vi "Target Vision Processing.vi"(4 "error in (no error)":errorcluster, 7 "Target Camera Image Size":T3=enum."160x120") -> ()   [LabVIEW 2015]
uses:
  Vision Support Code/Camera Types.ctl
  <vilib>/Rock Robotics/WPI/Camera/WPI_CameraImageSize.ctl
  <vilib>/Rock Robotics/WPI/Camera/WPI_CameraWhite Balance Values.ctl
  <vilib>/Rock Robotics/WPI/Camera/WPI_CameraExposure Values.ctl
  <vilib>/Rock Robotics/WPI/Camera/WPI_CameraFrameRate.ctl
  Robot Global Data.vi
  <vilib>/vision/NI_Vision_Development_Module.lvlib
panel:
  out "Highest Avg Score":dbl=93.76490466950331
  out "Detected Targets":T1(array[cluster])=[{"Distance (ft)"=10.934953821756244, "Center"={-0.006249999999999922, 0.175}, "Normalized Rect"={"Numeric"=-0.16249999999999998, "Numeric 2"=0.2833333333333333, "Numeric 3"=0.15000000000000013, "Numeric 5"=0.06666666666666665}}] {"Normalized Rect"."Numeric 5" format="%#_2g"; "Normalized Rect"."Numeric 3" format="%#_2g"; "Normalized Rect"."Numeric 2" format="%#_2g"; "Normalized Rect"."Numeric" format="%#_2g"}
  out "Sorted Particle Scores":T2(array[cluster])=[{"Rectangle px"={"Numeric"=67.0, "Numeric 2"=43.0, "Numeric 3"=92.0, "Numeric 5"=56.0}, "Aspect Ratio"=79.80769230769232, "Area to CH"=82.27848101265822, "X"=100.0, "Y"=100.0, "Moment Factor"=94.26815936617268}] {"Moment Factor" format="%#_3g"; "Aspect Ratio" format="%#_3g"; "Area to CH" format="%#_3g"; "X" format="%#_3g"; "Y" format="%#_3g"}
  in  "Display Original":bool=TRUE
  in  "Display Mask":bool=TRUE
  in  "Emphasize Limit Tests":bool=TRUE
  in  "Camera Type":T4=enum."MS HD3000 square"
  in  "Aspect Fudge Factor":dbl=1.0
  in  "Score Threshold":dbl=75.0
  out "Qualified Particles":i32=3
  in  "LED Color":T5={"Hue"={70.0, 10.0}, "Sat"={6.071428571428582, 255.0}, "Val"={127.5, 255.0}} {"Hue" scale=0.0..255.0 scale format="%#_3g"}
  out "Masked":T6(plugin-control)
  out "Original Image":T6(plugin-control)
  # "TARGET VISION PROCESSING.VI"
  # "This is only the initial camera size.\nOther camera setup is done\non the diagram. Notice it is set\nonce before the loop but can be\nupdated within the loop if needed."
  # "Origional Values\n--------------------------------------\nHue [10 -70]\nSat   [50 - 255]\nVal   [180 - 255]\nScore Threshold  [75]\nAspect Fudge Factor  [1]\nCamera Type  [MS HD3000 square]\nDisplay Origional  [OFF]\nDisplay Mask  [OFF]\nTarget Camera Image Size  [160x120]"
  # "Instructions:\nUse LED Color to threshold and build particles. Adjust calibration if needed.  Displays are very useful for debugging, but will slow down execution, so you may want to disable once working.\n\nAnnotations show the rectangle and the scores from top to bottom.  Change camera setting on diagram."
  # "Density Profile"
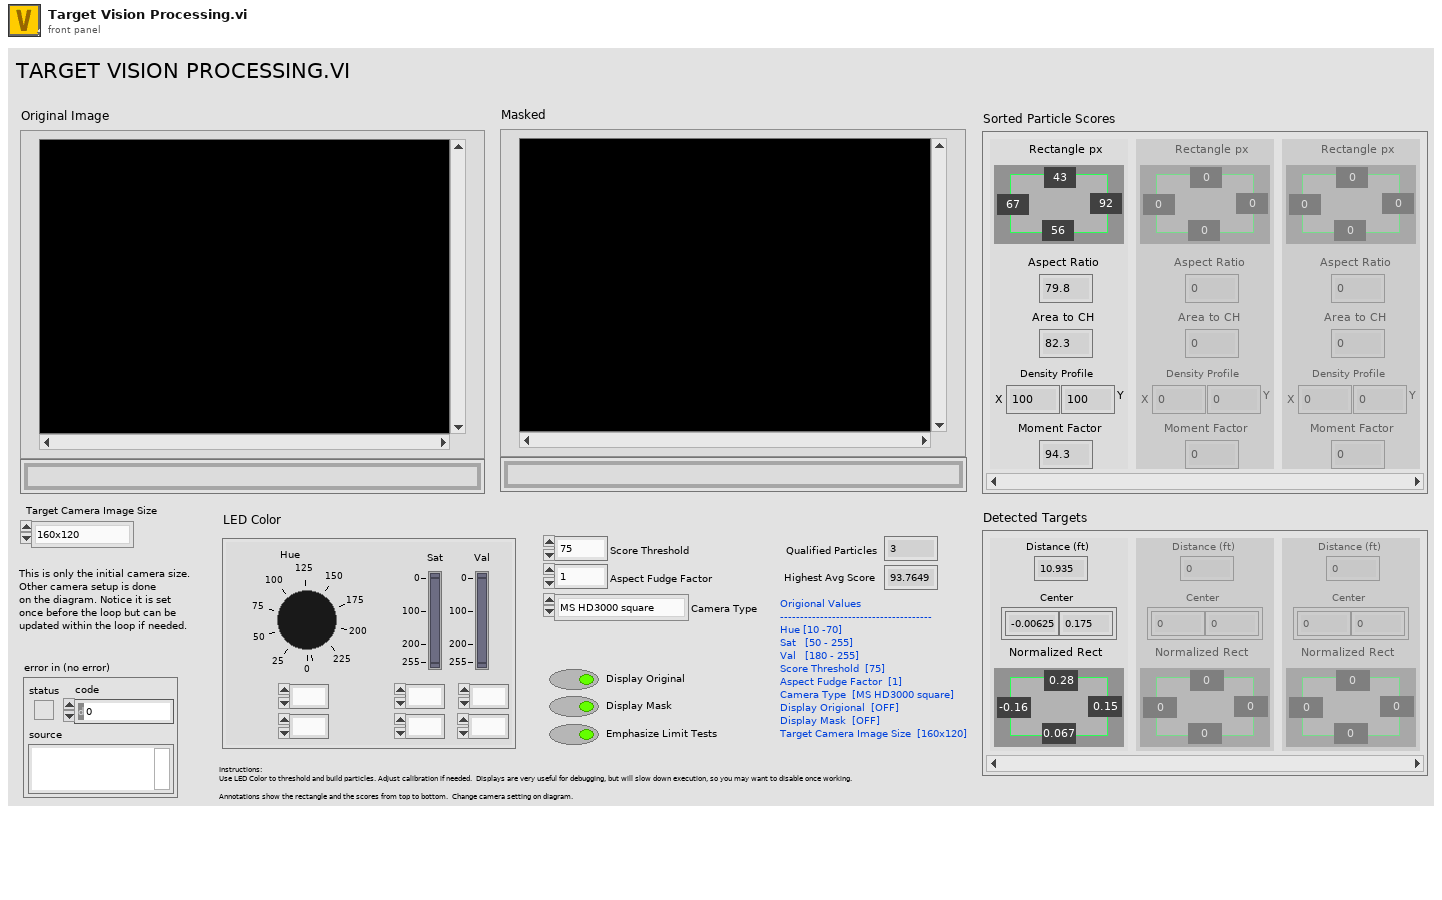
[diagram p1: front panel]
types:
  T1 = cluster{"Distance (ft)":dbl, "Center":cluster{dbl, dbl}, "Normalized Rect":cluster{"Numeric":dbl, "Numeric 2":dbl, "Numeric 3":dbl, "Numeric 5":dbl}}[]
  T2 = cluster{"Rectangle px":cluster{"Numeric":dbl, "Numeric 2":dbl, "Numeric 3":dbl, "Numeric 5":dbl}, "Aspect Ratio":dbl, "Area to CH":dbl, "X":dbl, "Y":dbl, "Moment Factor":dbl}[]
  T3 = typedef "WPI_CameraImageSize.ctl" = enum16{"640x480", "320x240", "160x120", "Custom"}
  T4 = typedef "Camera Types.ctl" = enum16{"206", "1011", "1013", "MS HD3000 square", "MS HD3000 640x480"}
  T5 = cluster{"Hue":cluster{dbl, dbl}, "Sat":cluster{dbl, dbl}, "Val":cluster{dbl, dbl}}
  T6 = typedef "IMAQ Image.ctl" = refnum<image>
  T7 = typedef "WPI_CameraFrameRate.ctl" = u32
  T8 = typedef "WPI_CameraExposure Values.ctl" = enum16{"Auto", "Flicker-free 50 Hz", "Flicker-free 60 Hz", "Hold current", "Custom"}
  T9 = typedef "WPI_CameraWhite Balance Values.ctl" = enum16{"Auto", "Fixed indoor", "Fixed outdoor 1", "Fixed outdoor 2", "Fixed fluorescent 1", "Fixed fluorescent 2", "Hold current", "Custom"}
  T10 = typedef "Particle Parameters" = i32
  T11 = typedef "Image Type" = u32
  T12 = typedef "WPI_CameraDevRef.ctl" = cluster{"Camera Address":string, "CameraStatus":errorcluster}
  T13 = cluster{"Bounding box":cluster{"left":dbl, "top":dbl, "right":dbl, "bottom":dbl}, "Aspect Ratio":dbl, "Area to CH":dbl, "X Mask":dbl, "Y Mask":dbl, "Moment":dbl}[]
  T14 = cluster{"Rectangle":cluster{"Numeric":dbl, "Numeric 2":dbl, "Numeric 3":dbl, "Numeric 5":dbl}, "L":dbl, "Area to CH":dbl, "X":dbl, "Y":dbl, "Moment Factor":dbl}[]
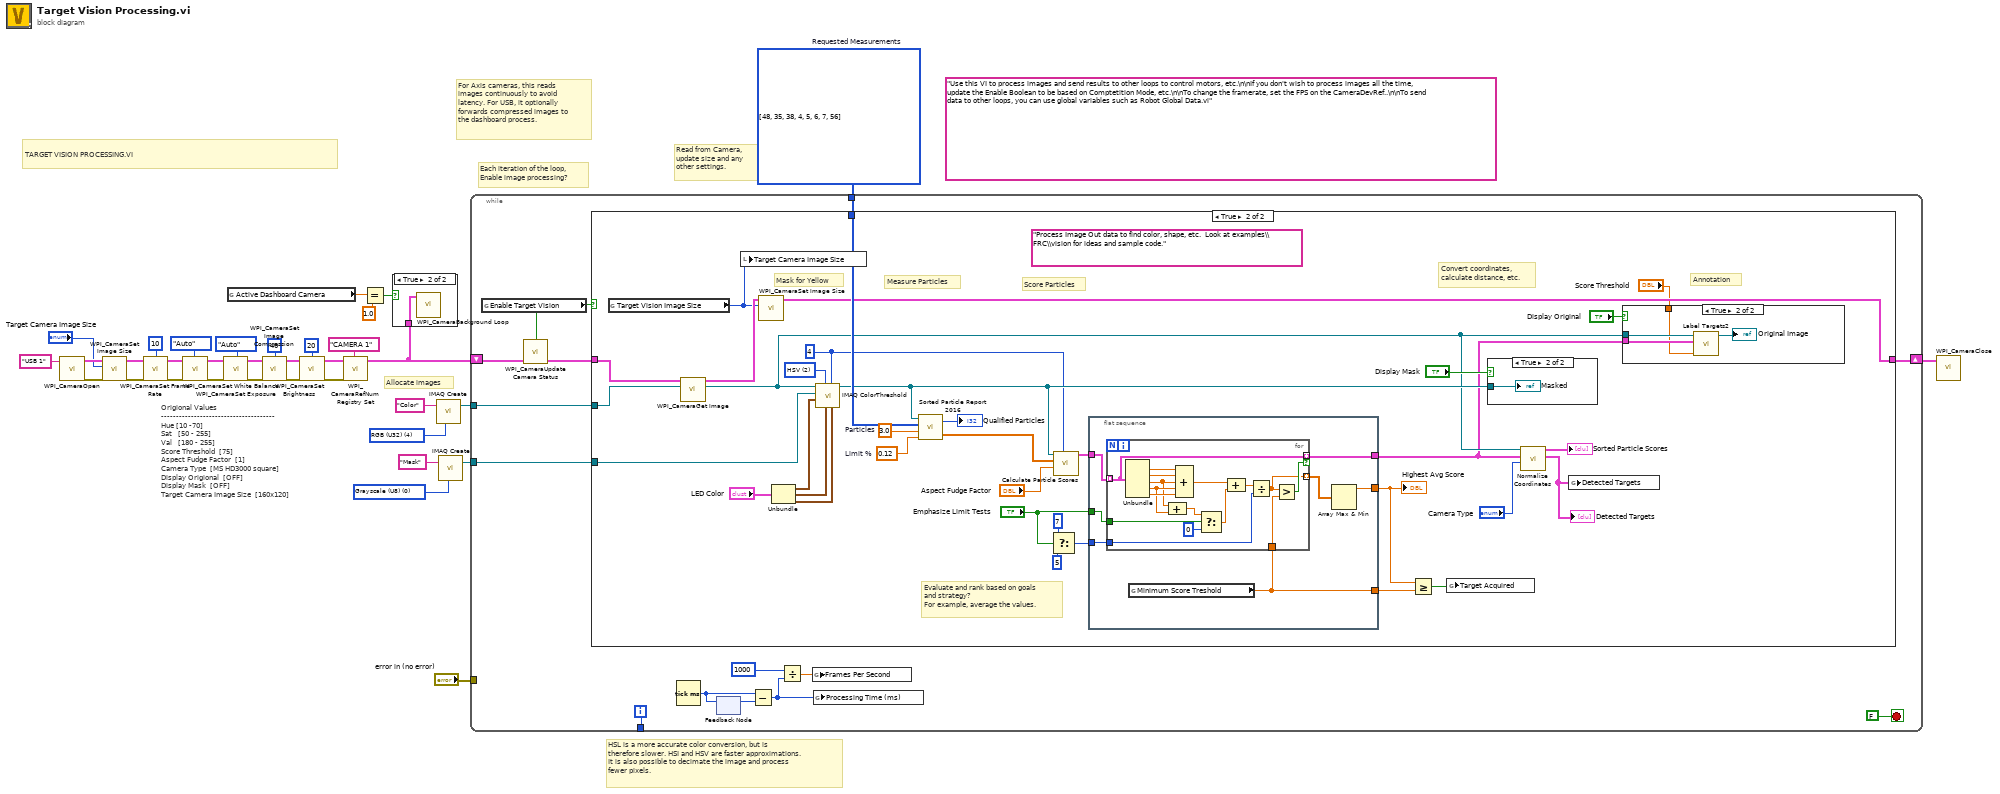
[diagram p0: block diagram]
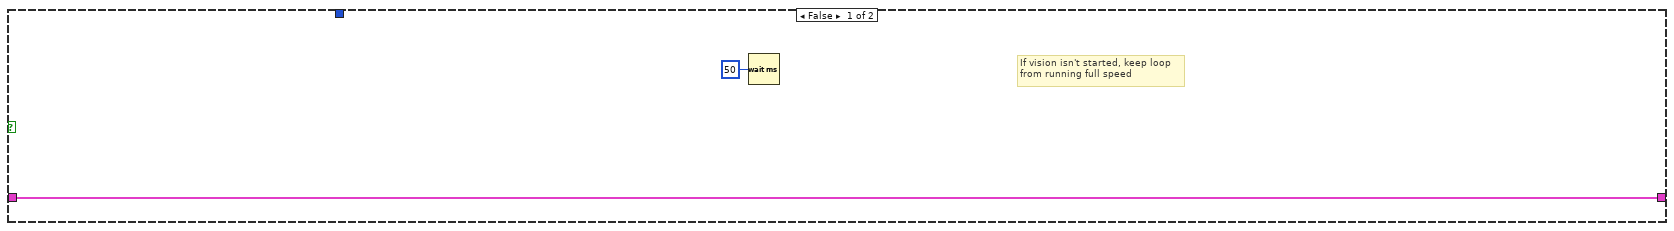
[diagram p3: hidden frame]
diagram:
  (unwired) "Use this VI to process images and send results to other loops to control motors, etc.\n\nIf you don't wish to process images all the time, update the Enable Boolean to be based on Comptetition Mode, etc.\n\nTo change the framerate, set the FPS on the CameraDevRef..\n\nTo send data to other loops, you can use global variables such as Robot Global Data.vi"
  w29 = T10[] [48, 35, 38, 4, 5, 6, 7, 56] items=["Center of Mass X", "Center of Mass Y", "First Pixel X", "First Pixel Y", "Bounding Rect Left", "Bounding Rect Top", "Bounding Rect Right", "Bounding Rect Bottom", "Max Feret Diameter Start X", "Max Feret Diameter Start Y", "Max Feret Diameter End X", "Max Feret Diameter End Y", "Max Horiz. Segment Length Left", "Max Horiz. Segment Length Right", "Max Horiz. Segment Length Row", "-", "Bounding Rect Width", "Bounding Rect Height", "Bounding Rect Diagonal", "Perimeter", "Convex Hull Perimeter", "Holes' Perimeter", "Max Feret Diameter", "Equivalent Ellipse Major Axis", "Equivalent Ellipse Minor Axis", "Equivalent Ellipse Minor Axis (Feret)", "Equivalent Rect Long Side", "Equivalent Rect Short Side", "Equivalent Rect Diagonal", "Equivalent Rect Short Side (Feret)", "Average Horiz. Segment Length", "Average Vert. Segment Length", "Hydraulic Radius", "Waddel Disk Diameter", "-", "Area", "Holes' Area", "Particle & Holes' Area", "Convex Hull Area", "Image Area", "-", "Number of Holes", "Number of Horiz. Segments", "Number of Vert. Segments", "-", "Orientation", "Max Feret Diameter Orientation", "-", "% Area/Image Area", "% Area/(Particle & Holes' Area)", "Ratio of Equivalent Ellipse Axes", "Ratio of Equivalent Rect Sides", "-", "Elongation Factor", "Compactness Factor", "Heywood Circularity Factor", "Type Factor", "-", "Sum X", "Sum Y", "Sum XX", "Sum XY", "Sum YY", "Sum XXX", "Sum XXY", "Sum XYY", "Sum YYY", "-", "Moment of Inertia XX", "Moment of Inertia XY", "Moment of Inertia YY", "Moment of Inertia XXX", "Moment of Inertia XXY", "Moment of Inertia XYY", "Moment of Inertia YYY", "Norm. Moment of Inertia XX", "Norm. Moment of Inertia XY", "Norm. Moment of Inertia YY", "Norm. Moment of Inertia XXX", "Norm. Moment of Inertia XXY", "Norm. Moment of Inertia XYY", "Norm. Moment of Inertia YYY", "Hu Moment 1", "Hu Moment 2", "Hu Moment 3", "Hu Moment 4", "Hu Moment 5", "Hu Moment 6", "Hu Moment 7"]  # Requested Measurements
  w32 = T11 0 items=["Grayscale (U8)", "Grayscale (I16)", "Grayscale (SGL)", "Complex (CSG)", "RGB (U32)", "HSL (U32)", "RGB (U64)", "Grayscale (U16)"] ("Image Type")
  w34 = T11 4 items=["Grayscale (U8)", "Grayscale (I16)", "Grayscale (SGL)", "Complex (CSG)", "RGB (U32)", "HSL (U32)", "RGB (U64)", "Grayscale (U16)"] ("Image Type")
  # "Origional Values\n--------------------------------------\nHue [10 -70]\nSat   [50 - 255]\nVal   [180 - 255]\nScore Threshold  [75]\nAspect Fudge Factor  [1]\nCamera Type  [MS HD3000 square]\nDisplay Origional  [OFF]\nDisplay Mask  [OFF]\nTarget Camera Image Size  [160x120]"
  # "TARGET VISION PROCESSING.VI"
  # "Read from Camera,\nupdate size and any\nother settings."
  # "Each iteration of the loop,\nEnable image processing?"
  # "HSL is a more accurate color conversion, but is\ntherefore slower. HSI and HSV are faster approximations.\nIt is also possible to decimate the image and process\nfewer pixels."
  # "For Axis cameras, this reads\nimages continuously to avoid\nlatency. For USB, it optionally\nforwards compressed images to\nthe dashboard process."
  # "Allocate images"
  n1 = call <vilib>:"WPI_CameraOpen.vi"("Camera Address"="USB 1" ("format string")) -> ("error out"=w19:errorcluster, "CameraDevRef"=w18:T12)  [unwired: 1 in, 8 out]
  n2 = call <vilib>:"WPI_CameraSet Image Size.vi"("error in (no error)"=w19, "Image Size"="Target Camera Image Size", "CameraDevRef"=w18) -> ("error out"=w20:errorcluster, "CameraDevRef Out"=w17:T12)  [unwired: 1 in, 6 out]
  n3 = call <vilib>:"WPI_CameraSet Frame Rate.vi"("error in (no error)"=w20, "Frame Rate (fps)"=T7 10, "CameraDevRef"=w17) -> ("error out"=w21:errorcluster, "CameraDevRef Out"=w15:T12)  [unwired: 7 out]
  n4 = call <vilib>:"WPI_CameraSet White Balance.vi"("error in (no error)"=w21, "White Balance"=WPI_CameraWhite_Balance_Values."Auto", "CameraDevRef"=w15) -> ("error out"=w22:errorcluster, "CameraDevRef Out"=w16:T12)  [unwired: 1 in, 6 out]
  n5 = call <vilib>:"WPI_CameraSet Exposure.vi"("error in (no error)"=w22, "Exposure"=WPI_CameraExposure_Values."Auto", "CameraDevRef"=w16) -> ("error out"=w23:errorcluster, "CameraDevRef Out"=w13:T12)  [unwired: 1 in, 6 out]
  n6 = global read "Robot Global Data.vi" "Active Dashboard Camera"() -> (w3:dbl)
  n7 = call <vilib>:"WPI_CameraSet Image Compression.vi"("error in (no error)"=w23, "Compression"=40, "CameraDevRef"=w13) -> ("error out"=w24:errorcluster, "CameraDevRef Out"=w14:T12)  [unwired: 7 out]
  n8 = call <vilib>:"WPI_CameraSet Brightness.vi"("error in (no error)"=w24, "Brightness"=20, "CameraDevRef"=w14) -> ("error out"=w25:errorcluster, "CameraDevRef Out"=w6:T12)  [unwired: 7 out]
  n9 = call <vilib>:"WPI_CameraRefNum Registry Set.vi"("error in (no error)"=w25, "refnum name"="CAMERA 1", "CameraDevRef"=w6) -> ("CameraDevRef"=w1:T12)  [unwired: 1 in, 7 out]
  n10 = Equal?(x=w3, y=1.0) -> (x = y?=w2:bool)
  n11 = case shown="True" w2 {
    tunnel: w1 -> [_ w36]
    frame False {
    }
    frame True {
      n12 = call <vilib>:"WPI_CameraBackground Loop.vi"("CameraDevRef"=w36) -> ()  [unwired: 11 in]
    }
  }
  n13 = call "IMAQ Create"("Image Name"="Color", "Image Type"=w34) -> ("New Image"=w33:T6)  [unwired: 2 in, 2 out]
  n14 = call "IMAQ Create"("Image Name"="Mask", "Image Type"=w32) -> ("New Image"=w30:T6)  [unwired: 2 in, 2 out]
  n15 = while {
    tunnel: w33 -> [w45]
    tunnel: w30 -> [w49]
    tunnel: w29 -> [w48]
    tunnel: "error in (no error)" -> [_]
    tunnel: [w44] -> _
    shift-right: [w42] -> w7
    shift-left: w1 -> [w39]
    i -> [w44]
    stop <- FALSE stop-if-true
    n16 = global read "Robot Global Data.vi" "Enable Target Vision"() -> (w37:bool)
    n17 = call <vilib>:"WPI_CameraUpdate Camera Status.vi"("CameraDevRef In"=w39, "Enable Vision"=w37) -> ("CameraDevRef Out"=w43:T12)  [unwired: 3 in]
    n18 = case shown="True" w37 {
      tunnel: w49 -> [_ w87]
      tunnel: w48 -> [_ w82]
      tunnel: w43 -> [w51 w79]
      tunnel: w45 -> [_ w78]
      tunnel: [w51 w76] -> w42
      frame False {
        # "If vision isn't started, keep loop\nfrom running full speed"
        n19 = Wait (ms)(milliseconds to wait=u32 50) -> ()  [unwired: 1 out]
      }
      frame True {
        w60 = 4 ("Replace Value")
        w73 = u16 2 items=["RGB", "HSL", "HSV", "HSI"] ("Color Mode")
        (unwired) "Process Image Out data to find color, shape, etc.  Look at examples\\FRC\\vision for ideas and sample code."
        w80 = 0.12  # Limit %
        w81 = 3.0  # Particles
        # "Evaluate and rank based on goals\nand strategy?\nFor example, average the values."
        # "Measure Particles"
        # "Convert coordinates,\ncalculate distance, etc."
        # "Annotation"
        # "Score Particles"
        # "Mask for Yellow"
        n20 = global read "Robot Global Data.vi" "Target Vision Image Size"() -> (w58:T3)
        n21 = call <vilib>:"WPI_CameraGet Image.vi"("Image"=w78, "CameraDevRef"=w79) -> ("Image Out"=w63:T6, "CameraDevRef Out"=w77:T12)  [unwired: 7 in, 1 out]
        n22 = local write "Target Camera Image Size"(w58) -> ()
        n23 = call <vilib>:"WPI_CameraSet Image Size.vi"("Image Size"=w58, "CameraDevRef"=w77) -> ("CameraDevRef Out"=w76:T12)  [unwired: 2 in, 7 out]
        n24 = Unbundle("LED Color") -> ("Hue"=w86:cluster{dbl, dbl}, "Sat"=w85:cluster{dbl, dbl}, "Val"=w84:cluster{dbl, dbl})
        n25 = call "IMAQ ColorThreshold"("Blue or Luma or Val or Inten Range"=w84, "Replace Value"=w60, "Green or Sat Range"=w85, "Color Mode"=w73, "Red or Hue Range"=w86, "Image Dst"=w87, "Image Src"=w63) -> ("Image Dst Out"=w72:T6)  [unwired: 3 in, 1 out]
        n26 = call "Sorted Particle Report 2016.vi"("Min Area Size %"=w80, "Particle Count Limit"=w81, "Pixel Measurements"=w82, "Image in"=w72) -> ("Sorted Data"=w71:dbl[][], "Particles"=→"Qualified Particles":i32)
        n27 = Select(t=7, s="Emphasize Limit Tests", f=5) -> (s? t:f=w66:i32)
        n28 = call "Calculate Particle Scores.vi"("Pixel Value"=w60, "Aspect Fudge Factor"="Aspect Fudge Factor", "Sorted Data"=w71, "Image in"=w72) -> ("Scores"=w69:T13)  [unwired: 7 in]
        n29 = flat-sequence {
          tunnel: w69 -> [w98]
          tunnel: w66 -> [w96]
          tunnel: [w99] -> w54
          tunnel: [w94] -> w62
          tunnel: "Emphasize Limit Tests" -> [w97]
          tunnel: [w93] -> w53
          frame #0 {
            n30 = global read "Robot Global Data.vi" "Minimum Score Treshold"() -> (w93:dbl)
            n31 = for {
              tunnel: w98 -> [w113] mode=indexing
              tunnel: [w113] -> w94 mode=indexing if=w112
              tunnel: [w111] -> w95 mode=indexing
              tunnel: w96 -> [w110]
              tunnel: w93 -> [w109]
              tunnel: w97 -> [w102]
              n32 = Unbundle(w113) -> ("Aspect Ratio"=w115:dbl, "Area to CH"=w114:dbl, "X Mask"=w104:dbl, "Y Mask"=w105:dbl, "Moment"=w106:dbl)  [unwired: 1 out]
              n33 = Compound Arithmetic op=ADD(w104, w105) -> (w103:dbl)
              n34 = Compound Arithmetic op=ADD(w115, w114, w104, w105, w106) -> (w108:dbl)
              n35 = Select(t=w103, s=w102, f=0) -> (s? t:f=w101:dbl)
              n36 = Compound Arithmetic op=ADD(w108, w101) -> (w107:dbl)
              n37 = Divide(x=w107, y=w110) -> (x/y=w111:dbl)
              n38 = Greater?(x=w111, y=w109) -> (0:w112:bool)
            }
            n39 = Array Max & Min(array=w95) -> (max value=w99:dbl)  [unwired: 3 out]
          }
        }
        n40 = Greater Or Equal?(x=w54, y=w53) -> (x >= y?=w55:bool)
        n41 = global write "Robot Global Data.vi" "Target Acquired"(w55) -> ()
        n42 = case shown="True" "Display Mask" {
          tunnel: w72 -> [_ w92]
          frame False {
          }
          frame True {
            "Masked" <- w92
          }
        }
        n43 = call "Normalize Coordinates.vi"("Camera Type"="Camera Type", "Targets"=w62, "Image in"=w63) -> ("Found Targets"=w59:T1, "Sorted Scores"=→"Sorted Particle Scores":T14)  [unwired: 7 in]
        "Detected Targets" <- w59
        n44 = global write "Robot Global Data.vi" "Detected Targets"(w59) -> ()
        n45 = case shown="True" "Display Original" {
          tunnel: w63 -> [_ w91]
          tunnel: w62 -> [_ w89]
          tunnel: "Score Threshold" -> [_ w88]
          frame False {
          }
          frame True {
            n46 = call "Label Targets2.vi"("Score Threshold"=w88, "Targets"=w89, "Image in"=w91) -> ("Image out"=→"Original Image":T6)  [unwired: 8 in]
          }
        }
        "Highest Avg Score" <- w54
      }
    }
    n47 = Tick Count (ms)() -> (millisecond timer value=w46:u32)
    n48 = feedback-in #1(w46) -> ()
    n49 = feedback #1() -> (w47:u32)  [unwired: 1 in]
    n50 = Subtract(x=w46, y=w47) -> (x-y=w41:u32)
    n51 = Divide(x=1000 ("Brightness"), y=w41) -> (x/y=w38:dbl)
    n52 = global write "Robot Global Data.vi" "Frames Per Second"(w38) -> ()
    n53 = global write "Robot Global Data.vi" "Processing Time (ms)"(w41) -> ()
  }
  n54 = call <vilib>:"WPI_CameraClose.vi"("CameraDevRef"=w7) -> ()  [unwired: 1 in, 10 out]
